vi "0mqManager.vi"(10 "intercomm configuration":T1) -> (0 "last error":errorcluster, 1 "exit":bool)   [LabVIEW 2018]
uses:
  Custom/S4msg.ctl
  <vilib>/addons/zeromq/socket_type.ctl
  <vilib>/addons/zeromq/zeromq.lvlib
  <vilib>/addons/zeromq/zmq_context.lvclass
  <vilib>/addons/zeromq/zmq_socket.lvclass
panel:
  out "endpointPULL":string="localhost"
  out "last tick":u32
  out "endpointPUB":string="localhost"
  out "S4ICS_status":string caption="Status received from S4ICS"
  out "S4ICS_command":string caption="Command sent to S4ICS"
  in  "Stop Client":bool
  # "S4ICS 0mqCOMM"
  # "COMMUNICATION CHANNEL"
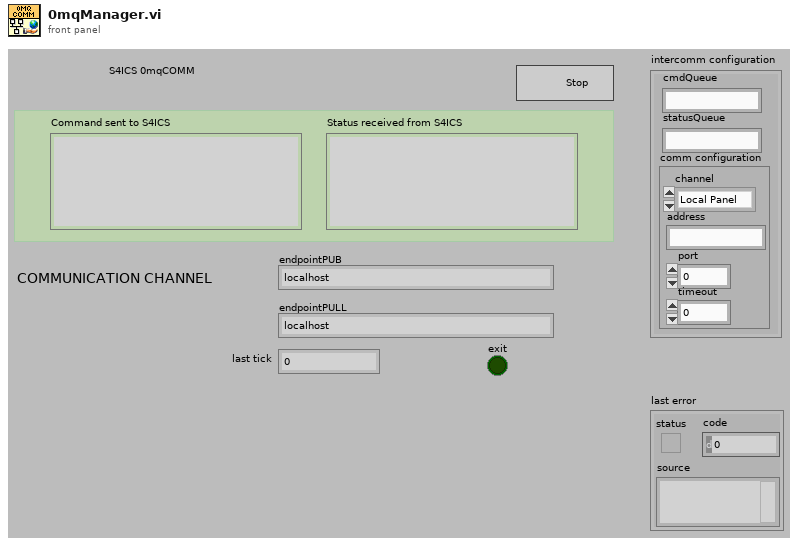
[diagram p1: front panel]
types:
  T1 = cluster{"S4commandQueueName":string, "S4statusQueueName":string, "comm configuration":cluster{"channel":enum32{"Local Panel", "Inner TCP/IP", "Outer TCP/IP", "MQTT", "ZeroMQ"}, "address":string, "port":u16, "timeout":i32}}
  T2 = typedef "zeromq.lvlib/socket_type.ctl" = enum8{"ZMQ_PAIR", "ZMQ_PUB", "ZMQ_SUB", "ZMQ_REQ", "ZMQ_REP", "ZMQ_DEALER", "ZMQ_ROUTER", "ZMQ_PULL", "ZMQ_PUSH", "ZMQ_XPUB", "ZMQ_XSUB", "ZMQ_STREAM", "ZMQ_SERVER", "ZMQ_CLIENT", "ZMQ_RADIO", "ZMQ_DISH", "ZMQ_GATHER", "ZMQ_SCATTER", "ZMQ_DGRAM"}
  T3 = typedef "S4msg.ctl" = cluster{"msg topic":string, "msg data":variant}
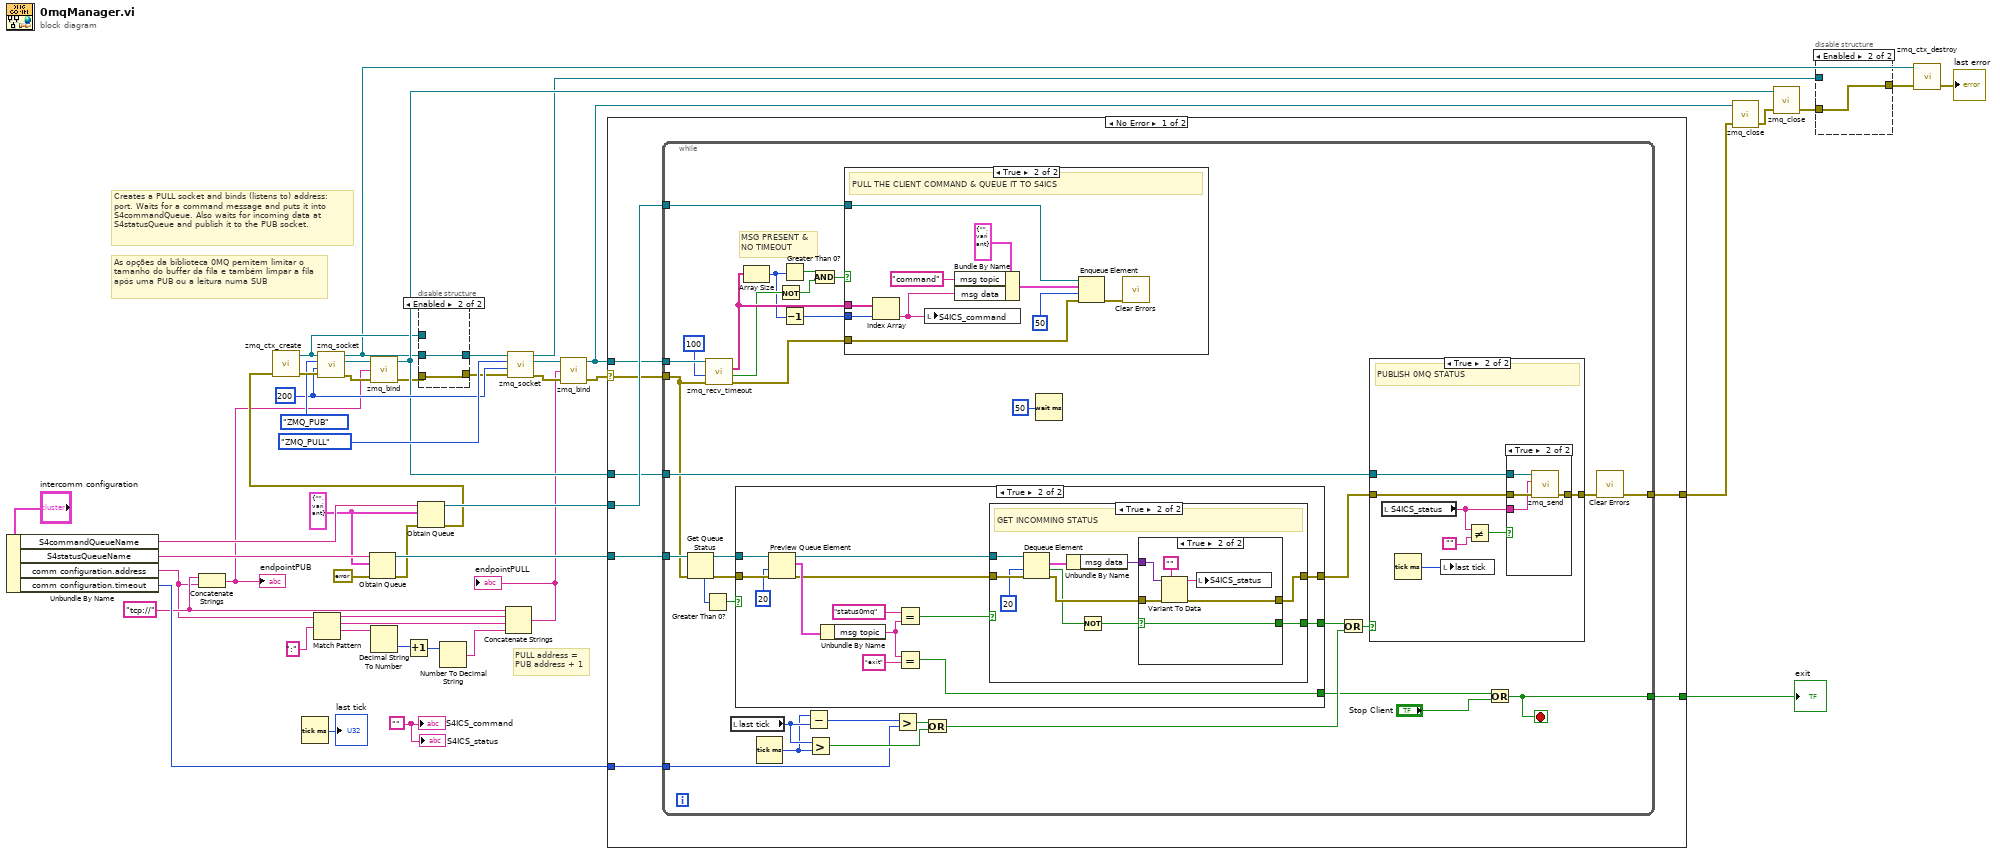
[diagram p0: block diagram]
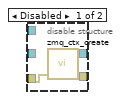
[diagram p2: hidden frame]
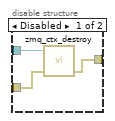
[diagram p3: hidden frame]
diagram:
  w3 = "tcp://"
  w24 = 200 ("linger (ms)")
  w38 = T3 {"msg topic"="", "msg data"=variant} ("S4msg")
  w46 = ""
  # "As opções da biblioteca 0MQ pemitem limitar o tamanho do buffer da fila e também limpar a fila após uma PUB ou a leitura numa SUB"
  # "PULL address =\nPUB address + 1"
  # "Creates a PULL socket and binds (listens to) address: port. Waits for a command message and puts it into S4commandQueue. Also waits for incoming data at S4statusQueue and publish it to the PUB socket."
  n1 = Unbundle By Name("intercomm configuration") -> ("S4commandQueueName"=w44:string, "S4statusQueueName"=w45:string, "comm configuration.address"=w1:string, "comm configuration.timeout"=w20:i32)
  n2 = Concatenate Strings(w3, w1) -> (w2:string)
  "endpointPUB" <- w2
  n3 = Tick Count (ms)() -> (millisecond timer value=→"last tick":u32)
  n4 = Match Pattern(string=w1, regular expression=":") -> (before substring=w26:string, match substring=w25:string, after substring=w5:string)  [unwired: 1 in, 1 out]
  n5 = Obtain Queue(name (unnamed)=w45, element data type=w38, error in (no error)=errorcluster {"status"=FALSE, "code"=0, "source"=""}) -> (queue out=w42:refnum<queue>, error out=w39:errorcluster)  [unwired: 2 in, 1 out]
  n6 = Decimal String To Number(string=w5) -> (number=w28:i32)  [unwired: 2 in, 1 out]
  n7 = Increment(x=w28) -> (x+1=w27:i32)
  n8 = Obtain Queue(name (unnamed)=w44, element data type=w38, error in (no error)=w39) -> (queue out=w43:refnum<queue>, error out=w41:errorcluster)  [unwired: 2 in, 1 out]
  n9 = call <vilib>:"zmq_ctx_create.vi"("error in"=w41) -> ("error out"=w36:errorcluster, "context out"=w7:refnum<class "zmq_context.lvclass">)  [unwired: 3 in]
  n10 = call <vilib>:"zmq_socket.vi"("error in"=w36, "linger (ms)"=w24, "socket type"=socket_type."ZMQ_PUB", "context in"=w7) -> ("error out"=w37:errorcluster, "socket out"=w34:refnum<class "zmq_socket.lvclass">, "context out"=w6:refnum<class "zmq_context.lvclass">)  [unwired: 1 in]
  n11 = call <vilib>:"zmq_bind.vi"("error in"=w37, "endpoint"=w2, "socket in"=w34) -> ("error out"=w11:errorcluster, "socket out"=w16:refnum<class "zmq_socket.lvclass">)  [unwired: 1 in]
  n12 = disable-structure shown="Enabled" {
    disable-tunnel: [w49 w50] -> w12
    disable-tunnel: w11 -> [w48 w51]
    disable-tunnel: [w47 w51] -> w10
    disable-tunnel: w7 -> [_ _]
    disable-tunnel: w6 -> [_ w50]
    frame Disabled {
      n13 = call <vilib>:"zmq_ctx_create.vi"("error in"=w48) -> ("error out"=w47:errorcluster, "context out"=w49:refnum<class "zmq_context.lvclass">)  [unwired: 3 in]
    }
    frame Enabled {
    }
  }
  n14 = Number To Decimal String(number=w27) -> (decimal integer string=w4:string)  [unwired: 1 in]
  n15 = Concatenate Strings(w3, w26, w25, w4) -> (w9:string)
  "endpointPULL" <- w9
  n16 = call <vilib>:"zmq_socket.vi"("error in"=w10, "linger (ms)"=w24, "socket type"=socket_type."ZMQ_PULL", "context in"=w12) -> ("error out"=w33:errorcluster, "socket out"=w31:refnum<class "zmq_socket.lvclass">, "context out"=w14:refnum<class "zmq_context.lvclass">)  [unwired: 1 in]
  n17 = call <vilib>:"zmq_bind.vi"("error in"=w33, "endpoint"=w9, "socket in"=w31) -> ("error out"=w23:errorcluster, "socket out"=w21:refnum<class "zmq_socket.lvclass">)  [unwired: 1 in]
  n18 = case shown="No Error" w23 {
    selector: w23 -> [w55 w152]
    tunnel: w43 -> [w59 _]
    tunnel: w42 -> [w58 _]
    tunnel: w21 -> [w57 _]
    tunnel: w16 -> [w56 _]
    tunnel: [w54 w152] -> w22
    tunnel: w20 -> [w53 _]
    tunnel: [w52 _] -> w8
    frame No Error {
      n19 = while {
        tunnel: [w69] -> w54
        tunnel: w59 -> [w74]
        tunnel: w58 -> [w93]
        tunnel: w57 -> [w81]
        tunnel: w56 -> [w85]
        tunnel: w55 -> [w70]
        tunnel: w53 -> [w67]
        tunnel: [w62] -> w52
        stop <- w62 stop-if-true
        # "MSG PRESENT &\nNO TIMEOUT"
        n20 = Get Queue Status(queue=w93, error in (no error)=w70) -> (queue out=w66:refnum<queue>, error out=w65:errorcluster, # elements in queue=w63:i32)  [unwired: 1 in, 5 out]
        n21 = Greater Than 0?(x=w63) -> (x > 0?=w64:bool)
        n22 = call <vilib>:"zmq_recv_timeout.vi"("error in"=w70, "timeout (ms)"=u32 100, "socket in"=w81) -> ("error out"=w73:errorcluster, "timeout?"=w76:bool, "parts"=w79:string[])  [unwired: 1 in, 1 out]
        n23 = local read "last tick"() -> (w91:u32)
        n24 = case shown="True" w64 {
          selector: w64 -> [w94 _]
          tunnel: [w95 w108] -> w84
          tunnel: [w94 w107] -> w82
          tunnel: [w94 w96] -> w68
          tunnel: w66 -> [_ w106]
          tunnel: w65 -> [w95 w105]
          frame False {
          }
          frame True {
            n25 = Preview Queue Element(queue=w106, timeout in ms (-1)=20, error in (no error)=w105) -> (queue out=w101:refnum<queue>, element=w104:T3, error out=w100:errorcluster)  [unwired: 1 out]
            n26 = Unbundle By Name(w104) -> ("msg topic"=w97:string)
            n27 = Equal?(x="status0mq" ("msg topic"), y=w97) -> (x = y?=w102:bool)
            n28 = Equal?(x=w97, y="exit" ("msg topic")) -> (x = y?=w96:bool)
            n29 = case shown="True" w102 {
              selector: w102 -> [w109 _]
              tunnel: w100 -> [w110 w120]
              tunnel: w101 -> [_ w119]
              tunnel: [w110 w115] -> w108
              tunnel: [w109 w111] -> w107
              frame False {
              }
              frame True {
                # "GET INCOMMING STATUS"
                n30 = Dequeue Element(queue=w119, timeout in ms (-1)=20, error in (no error)=w120) -> (element=w118:T3, timed out?=w113:bool, error out=w116:errorcluster)  [unwired: 1 out]
                n31 = Unbundle By Name(w118) -> ("msg data"=w117:variant)
                n32 = Not(x=w113) -> (.not. x?=w112:bool)
                n33 = case shown="True" w112 {
                  selector: w112 -> [w122 w123]
                  tunnel: w117 -> [_ w128]
                  tunnel: w116 -> [w121 w127]
                  tunnel: [w121 w126] -> w115
                  tunnel: [w122 w123] -> w111
                  frame False {
                  }
                  frame True {
                    n34 = Variant To Data(error in=w127, type="", Variant=w128) -> (data=w124:string, error out=w126:errorcluster)
                    n35 = local write "S4ICS_status"(w124) -> ()
                  }
                }
              }
            }
          }
        }
        n36 = Array Size(array=w79) -> (size(s)=w72:i32)
        n37 = Tick Count (ms)() -> (millisecond timer value=w90:u32)
        n38 = Not(x=w76) -> (.not. x?=w77:bool)
        n39 = Greater Than 0?(x=w72) -> (x > 0?=w78:bool)
        n40 = Decrement(x=w72) -> (x-1=w71:i32)
        n41 = Subtract(x=w90, y=w91) -> (x-y=w92:u32)
        n42 = Greater?(x=w91, y=w90) -> (0:w88:bool)
        n43 = And(x=w78, y=w77) -> (x .and. y?=w75:bool)
        n44 = case shown="True" w75 {
          tunnel: w79 -> [_ w137]
          tunnel: w74 -> [_ w132]
          tunnel: w73 -> [_ w131]
          tunnel: w71 -> [_ w130]
          frame False {
          }
          frame True {
            # "PULL THE CLIENT COMMAND & QUEUE IT TO S4ICS"
            n45 = Index Array(array=w137, index=w130) -> (element=w134:string)
            n46 = local write "S4ICS_command"(w134) -> ()
            n47 = Bundle By Name(cluster=T3 {"msg topic"="", "msg data"=variant} ("S4msg"), "msg topic"="command", "msg data"=w134) -> (w133:T3)
            n48 = Enqueue Element(queue=w132, element=w133, timeout in ms (-1)=50, error in (no error)=w131) -> (error out=w129:errorcluster)  [unwired: 2 out]
            n49 = call <vilib>:"Clear Errors.vi"("error in (no error)"=w129) -> ()  [unwired: 5 in, 2 out]
          }
        }
        n50 = Greater?(x=w92, y=w67) -> (0:w89:bool)
        n51 = Or(x=w89, y=w88) -> (x .or. y?=w87:bool)
        n52 = Wait (ms)(milliseconds to wait=u32 50) -> ()  [unwired: 1 out]
        n53 = Or(x=w82, y=w87) -> (x .or. y?=w86:bool)
        n54 = case shown="True" w86 {
          tunnel: [w139 w143] -> w83
          tunnel: w85 -> [_ w146]
          tunnel: w84 -> [w139 w145]
          frame False {
          }
          frame True {
            # "PUBLISH 0MQ STATUS"
            n55 = local read "S4ICS_status"() -> (w140:string)
            n56 = Tick Count (ms)() -> (millisecond timer value=w144:u32)
            n57 = local write "last tick"(w144) -> ()
            n58 = Not Equal?(x=w140, y="") -> (x != y?=w141:bool)
            n59 = case shown="True" w141 {
              tunnel: w146 -> [_ w151]
              tunnel: w145 -> [w147 w150]
              tunnel: [w147 w149] -> w143
              tunnel: w140 -> [_ w148]
              frame False {
              }
              frame True {
                n60 = call <vilib>:"zmq_send.vi"("error in"=w150, "data"=w148, "socket in"=w151) -> ("error out"=w149:errorcluster)  [unwired: 4 in, 1 out]
              }
            }
          }
        }
        n61 = Or(x=w68, y="Stop Client") -> (x .or. y?=w62:bool)
        n62 = call <vilib>:"Clear Errors.vi"("error in (no error)"=w83) -> ("error out"=w69:errorcluster)  [unwired: 5 in, 1 out]
      }
    }
    frame Error {
    }
  }
  "exit" <- w8
  n63 = call <vilib>:"zmq_close.vi"("error in"=w22, "socket"=w21) -> ("error out"=w18:errorcluster)  [unwired: 3 in]
  n64 = call <vilib>:"zmq_close.vi"("error in"=w18, "socket"=w16) -> ("error out"=w17:errorcluster)  [unwired: 3 in]
  n65 = disable-structure shown="Enabled" {
    disable-tunnel: w17 -> [w155 w156]
    disable-tunnel: [w154 w156] -> w15
    disable-tunnel: w14 -> [w153 _]
    frame Disabled {
      n66 = call <vilib>:"zmq_ctx_destroy.vi"("error in"=w155, "context in"=w153) -> ("error out"=w154:errorcluster)  [unwired: 3 in]
    }
    frame Enabled {
    }
  }
  n67 = call <vilib>:"zmq_ctx_destroy.vi"("error in"=w15, "context in"=w6) -> ("error out"=→"last error":errorcluster)  [unwired: 3 in]
  "S4ICS_command" <- w46
  "S4ICS_status" <- w46
